vi "1.0_plus.vi"() -> ()   [LabVIEW 2019]
panel:
  out "숫자형":dbl
  in  "탱크2":dbl(slide) scale=0.0..10.0
  in  "탱크1":dbl(slide) scale=0.0..10.0
  out "탱크 3":dbl(slide) scale=0.0..50.0
  out "출력 1":dbl
  out "출력 4":dbl
  out "출력 3":dbl
  in  "입력 2":dbl
  in  "입력 1":dbl
  out "출력 2":dbl
  # "-"
  # "+"
  # "="
  # "/"
  # "x"
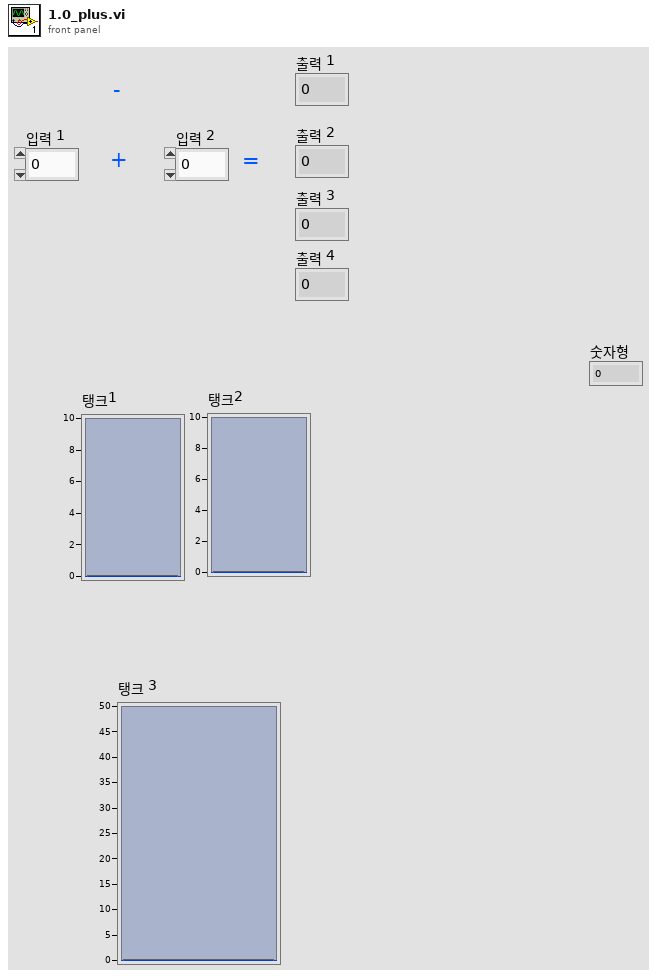
[diagram p1: front panel]
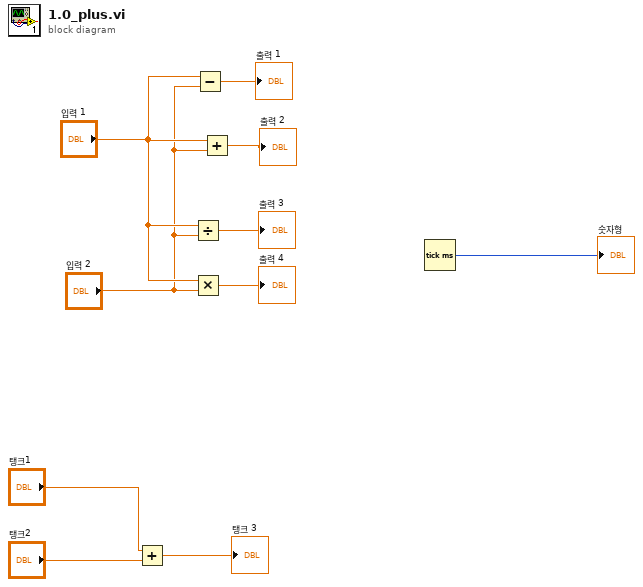
[diagram p0: block diagram]
diagram:
  n1 = Add(x="탱크1", y="탱크2") -> (x+y=→"탱크 3":dbl)
  n2 = Divide(x="입력 1", y="입력 2") -> (x/y=→"출력 3":dbl)
  n3 = Multiply(x="입력 1", y="입력 2") -> (x*y=→"출력 4":dbl)
  n4 = Subtract(x="입력 1", y="입력 2") -> (x-y=→"출력 1":dbl)
  n5 = Add(x="입력 1", y="입력 2") -> (x+y=→"출력 2":dbl)
  n6 = Tick Count (ms)() -> (millisecond timer value=→"숫자형":u32)
